vi "HEWH RLT Process Agilent Data.vi"(0 "Data Array":string[][](array[string]), 5 "Labels, Agilent":string[](array[string]), 7 "Agilent Data":dbl[](array[numeric])) -> (4 "Appended Data Array":string[][](array[string]), 8 "Data array w/ subset deleted":dbl[](array[numeric]))   [LabVIEW 2014]
panel:
  # "Assumes that the Labels correspond with the first elements in the data, and appends\nthe 2d Label/Data array to the input array.  Outputs the data array with the data removed that is used in \nthe output 2d string array."
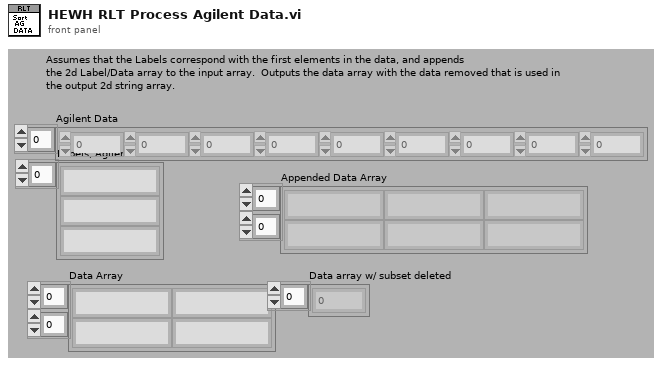
[diagram p1: front panel]
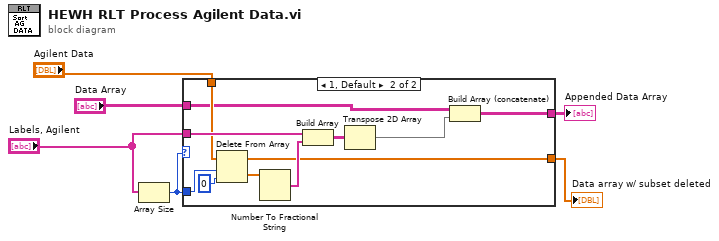
[diagram p0: block diagram]
diagram:
  n1 = Array Size(array="Labels, Agilent") -> (size(s)=w6:i32)
  n2 = case shown="1, Default" w6 {
    tunnel: "Labels, Agilent" -> [_ w19]
    tunnel: w6 -> [_ w17]
    tunnel: "Agilent Data" -> [w7 w15]
    tunnel: "Data Array" -> [w8 w11]
    tunnel: [w8 w10] -> w2
    tunnel: [w7 w12] -> w1
    frame 0 {
    }
    frame 1, Default {
      n3 = Delete From Array(array=w15, length=w17, index=0) -> (deleted portion=w18:dbl[], array with subset deleted=w12:dbl[])
      n4 = Number To Fractional String(number=w18) -> (F-format string=w16:string[])  [unwired: 3 in]
      n5 = Build Array(w19, w16) -> (w14:string[][])
      n6 = Transpose 2D Array(2D array=w14) -> (transposed array=w13:string[][])
      n7 = Build Array (concatenate)(w11, w13) -> (w10:string[][])
    }
  }
  "Appended Data Array" <- w2
  "Data array w/ subset deleted" <- w1
